vi "Obtain Trend.vi"(10 "Trend Count":dbl, 11 "Data In":T1) -> (3 "Array":dbl[](array[numeric]))   [LabVIEW 2015, in "XTrend.xctl"]
uses:
  XTrend.xctl
  XTrend_Data.ctl
  <vilib>/Analysis/baseanly.llb/Mean (DBL).vi
  <vilib>/Analysis/NI_AALBase.lvlib
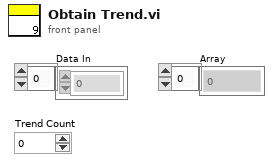
[diagram p1: front panel]
types:
  T1 = typedef "XTrend.xctl/XTrend_Data.ctl" = dbl[]
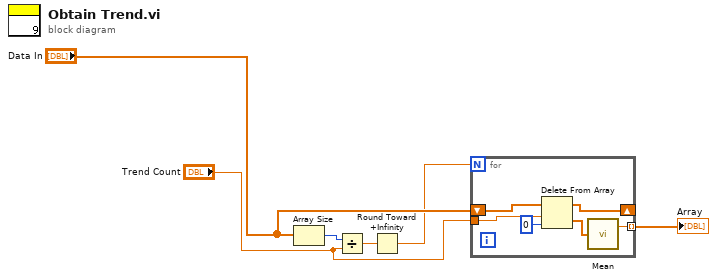
[diagram p0: block diagram]
diagram:
  n1 = Array Size(array="Data In") -> (size(s)=w1:i32)
  n2 = Divide(x=w1, y="Trend Count") -> (x/y=w2:dbl)
  n3 = Round Toward +Infinity(x=w2) -> (ceil(x): smallest int >= x=w3:dbl)
  n4 = for {
    N: w3 -> [_]
    tunnel: "Trend Count" -> [w11]
    shift-right: [w9] -> _
    shift-left: "Data In" -> [w12]
    tunnel: [w7] -> w6 mode=indexing
    n5 = Delete From Array(array=w12, length=w11, index=0) -> (deleted portion=w8:T1, array with subset deleted=w9:T1)
    n6 = call-poly <vilib>:"Mean.vi"("X"=w8) -> ("mean"=w7:dbl)  [unwired: 1 out]
  }
  "Array" <- w6
